vi "Rotary Condensentrator.vi"(7 "Speed Upgrades":u32 max=8, 11 "Liquid (mB/t)":u32) -> (0 "Limiting":bool, 3 "Gas (mB/t)":u32)   [LabVIEW 2023]
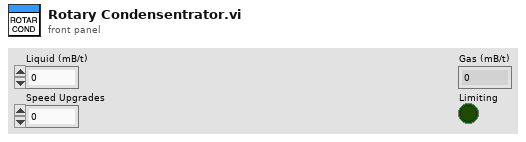
[diagram p1: front panel]
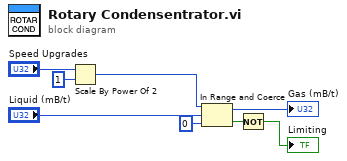
[diagram p0: block diagram]
diagram:
  n1 = Scale By Power Of 2(n="Speed Upgrades", x=u32 1) -> (x*2^n=w5:u32)
  n2 = In Range and Coerce(upper limit=w5, x="Liquid (mB/t)", lower limit=u32 0) -> (coerced(x)=→"Gas (mB/t)":u32, In Range?=w2:bool)
  n3 = Not(x=w2) -> (.not. x?=→"Limiting":bool)
